vi "State Exit Core.vi"(8 "error in (no error)":errorcluster, 11 "B Context State in":refnum<class "B Context State.lvclass">) -> (0 "error out":errorcluster, 3 "B Context State out":refnum<class "B Context State.lvclass">)   [LabVIEW 2021, in "B Context State.lvclass"]
uses:
  B Context State.lvclass
  B Context State.lvclass/B Context State.ctl
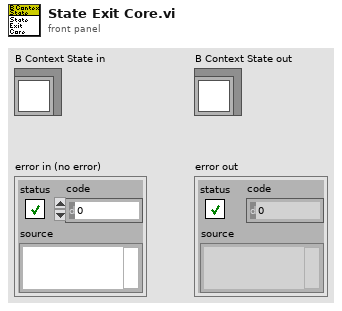
[diagram p1: front panel]
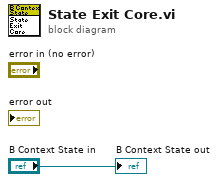
[diagram p0: block diagram]
diagram:
  "B Context State out" <- "B Context State in"
